vi "FPGA Host.vi"() -> ()   [LabVIEW 2009]
uses:
  <vilib>/rvi/DataTransferAndStorage/Container/XNode/niFpgaContainer.xnode
  <vilib>/rvi/interface/RandomDataEmulation/niFpgaRandomDataHandleErrors.vi
  <vilib>/rvi/interface/RandomDataEmulation/nirviRandomDataFPGAFIFO.vi
  <vilib>/rvi/DataTransferAndStorage/Container/Common/niFpgaContainerMethod.ctl
  <vilib>/rvi/DataTransferAndStorage/Container/Common/niFpgaTransferTypeControl.ctl
panel:
  out "Target to Host Timed Out?":bool
  out "Host to Target Timed Out?":bool
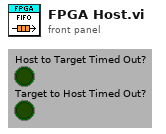
[diagram p1: front panel]
types:
  T1 = typedef "niFpgaContainerMethod.ctl" = enum16{"Write", "Read", "Clear", "Get Number of Elements to Write", "Get Number of Elements to Read", "Enable", "Disable", "Flush and Disable", "Get Stream State"}
  T2 = typedef "niFpgaTransferTypeControl.ctl" = enum16{"Target-Scoped", "Host to Target - DMA", "Target to Host - DMA", "Peer to Peer Reader", "Peer to Peer Writer", "Bidirectional"}
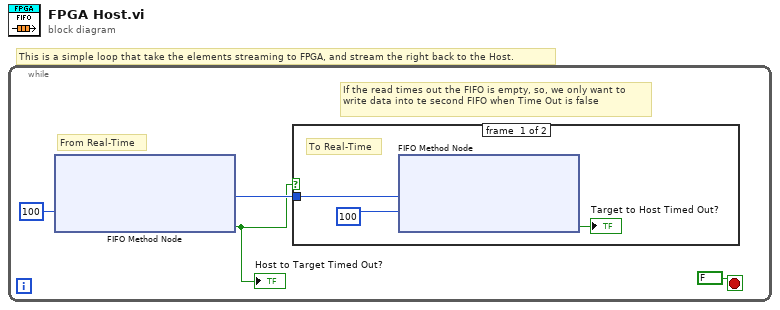
[diagram p0: block diagram]
diagram:
  # "This is a simple loop that take the elements streaming to FPGA, and stream the right back to the Host."
  n1 = while {
    stop <- FALSE stop-if-true
    # "From Real-Time"
    # "If the read times out the FIFO is empty, so, we only want to write data into te second FIFO when Time Out is false"
    n2 = xnode ("FIFO Method Node")("Timeout"=100) -> ("Element"=w4:i16, "Timed Out?"=w1:bool)  [unwired: 1 in, 1 out]
    "Host to Target Timed Out?" <- w1
    n3 = case shown="False" w1 {
      tunnel: w4 -> [w7 _]
      frame #0 {
        # "To Real-Time"
        n4 = xnode ("FIFO Method Node")("Element"=w7, "Timeout"=100) -> ("Timed Out?"=→"Target to Host Timed Out?":bool)  [unwired: 1 in, 1 out]
      }
      frame #1 {
      }
    }
  }
